vi "DAQmx.Create Sample Clock.vi"(8 "error in (no error)":errorcluster, 11 "DAQmx in":refnum<class "DAQmx.lvclass">) -> (0 "error out":errorcluster, 3 "DAQmx out":refnum<class "DAQmx.lvclass">)   [LabVIEW 2019, in "DAQmx.lvclass"]
uses:
  DAQmx.lvclass
  typedefs/DAQ.Config.Timing.Sampling--Cluster.ctl
  DAQmx.lvclass/DAQmx.ctl
  <vilib>/DAQmx/configure/timing.llb/DAQmx Timing (Sample Clock).vi
  <resource>/objmgr/daqmx.rc
panel:
  out "SampClk.Rate":dbl
  out "Sampling":T1={"Fs"=204789.0, "#s"=15753} {"Fs" format="%#_13g"}
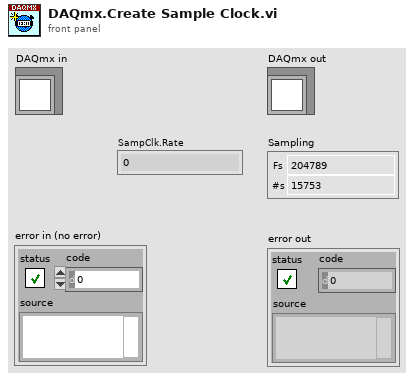
[diagram p1: front panel]
types:
  T1 = typedef "DAQmx.lvclass/DAQ.Config.Timing.Sampling--Cluster.ctl" = cluster{"Fs":dbl, "#s":i32}
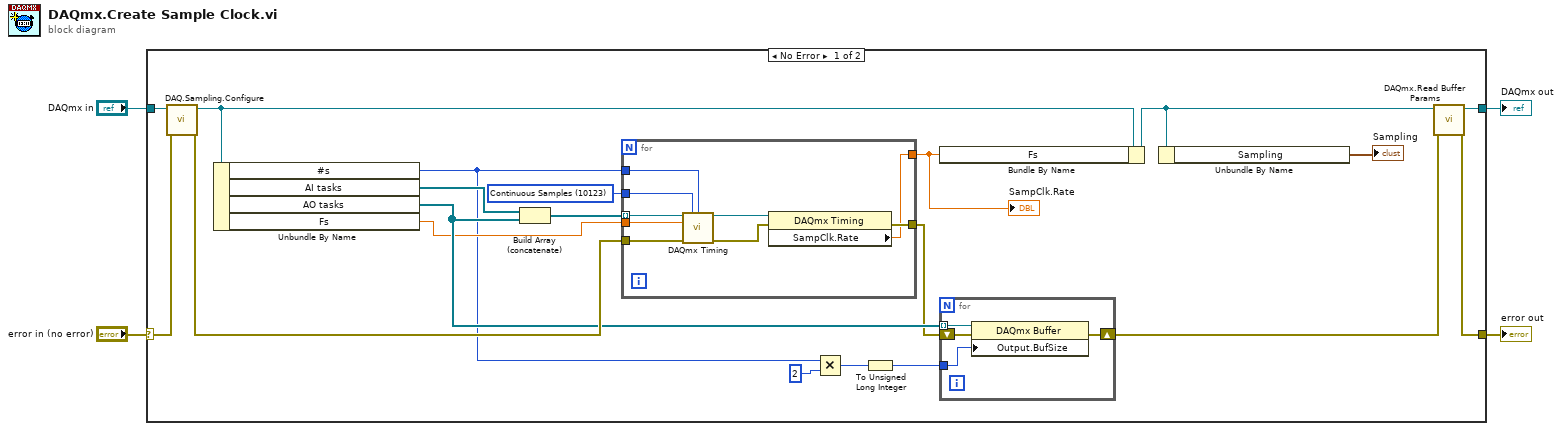
[diagram p0: block diagram]
diagram:
  n1 = case shown="No Error" "error in (no error)" {
    selector: "error in (no error)" -> [w19 w39]
    tunnel: [w7 w39] -> w4
    tunnel: [w8 w38] -> w2
    tunnel: "DAQmx in" -> [w24 w38]
    frame No Error {
      w18 = 10123 items=["Finite Samples"=10178, "Continuous Samples"=10123, "Hardware Timed Single Point"=12522] ("sample mode")
      n2 = call "DAQ.Sampling.Configure.vi"("error in (no error)"=w19, "DAQmx in"=w24) -> ("error out"=w22:errorcluster, "DAQmx out"=w23:refnum<class "DAQmx.lvclass">)  [unwired: 7 in, 1 out]
      n3 = Unbundle By Name(w23) -> ("#s"=w14:i32, "AI tasks"=w20:refnum<k21>[], "AO tasks"=w17:refnum<k21>[], "Fs"=w15:dbl)
      n4 = Build Array (concatenate)(w20, w17) -> (w21:refnum<k21>[])
      n5 = for {
        tunnel: w21 -> [w29] mode=indexing
        tunnel: w15 -> [w28]
        tunnel: w22 -> [w27]
        tunnel: [w31] -> w10
        tunnel: [w25] -> w5
        tunnel: w14 -> [w30]
        tunnel: w18 -> [w26]
        n6 = call-poly <vilib>:"DAQmx Timing.vi"("task/channels in"=w29, "sample mode"=w26, "samples per channel"=w30, "rate"=w28, "error in"=w27) -> ("task out"=w33:refnum<k21>, "error out"=w32:errorcluster)  [unwired: 9 in]
        n7 = property class="DAQmx Timing"(reference=w33, error in=w32) -> (error out=w31:errorcluster, "SampClk.Rate"=w25:dbl)  [unwired: 1 out]
      }
      "SampClk.Rate" <- w5
      n8 = Multiply(x=w14, y=2) -> (x*y=w12:i32)
      n9 = To Unsigned Long Integer(number=w12) -> (unsigned 32bit integer=w11:u32)
      n10 = Bundle By Name(cluster=w23, "Fs"=w5) -> (w9:refnum<class "DAQmx.lvclass">)
      n11 = for {
        tunnel: w17 -> [w37] mode=indexing
        tunnel: w11 -> [w36]
        shift-right: [w34] -> w6
        shift-left: w10 -> [w35]
        n12 = property class="DAQmx Buffer"(reference=w37, error in=w35, "Output.BufSize"=w36) -> (error out=w34:errorcluster)  [unwired: 1 out]
      }
      n13 = Unbundle By Name(w9) -> ("Sampling"=→"Sampling":T1)
      n14 = call "DAQmx.Read Buffer Params.vi"("error in (no error)"=w6, "DAQmx in"=w9) -> ("error out"=w7:errorcluster, "DAQmx out"=w8:refnum<class "DAQmx.lvclass">)  [unwired: 8 in]
    }
    frame Error {
    }
  }
  "error out" <- w4
  "DAQmx out" <- w2
